vi "XML.Memory.Load.vi"(8 "error in (no error)":errorcluster, 11 "XML file path":path) -> (0 "error out":errorcluster, 2 "all parameter names":string[](array[string]), 3 "Data Value Reference out":refnum<data-value>)   [LabVIEW 2019, in "Tools.lvlib"]
uses:
  Tools.lvlib
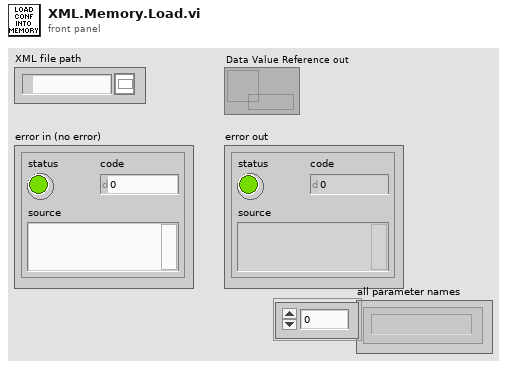
[diagram p1: front panel]
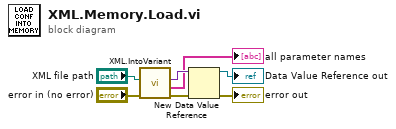
[diagram p0: block diagram]
diagram:
  n1 = call "XML.IntoVariant.vi"("error in"="error in (no error)", "XML file path"="XML file path") -> ("error out"=w4:errorcluster, "all parameter names"=→"all parameter names":string[], "variant"=w2:variant)  [unwired: 7 in]
  n2 = New Data Value Reference(data value=w2, error in=w4) -> (data value reference=→"Data Value Reference out":refnum<data-value>, error out=→"error out":errorcluster)
